vi "RT_I2C Configure.vi"(7 "Address Type (7-bit)":enum16{"7-bit", "10-bit"}(ring), 8 "error in":errorcluster, 9 "Clock Rate":u32, 10 "IICSlaveAddress":u16, 11 "FPGA VI Reference In":T1) -> (0 "error out":errorcluster, 3 "FPGA VI Reference Out":T1)   [LabVIEW 2018]
uses:
  Data Def/RT_FPGA VI Reference.ctl
  <vilib>/Utility/error.llb/Error Cluster From Error Code.vi
  <vilib>/rvi/errors/niLvFpgaAdjustHostInterfaceError.vi
  <vilib>/rvi/interface/nirviReadWriteControl/nirviReadWriteControl.xnode
  NiFpgaLv.dll
  <vilib>/rvi/interface/Simulation/niFpgaSimulationCallBeginRW.vi
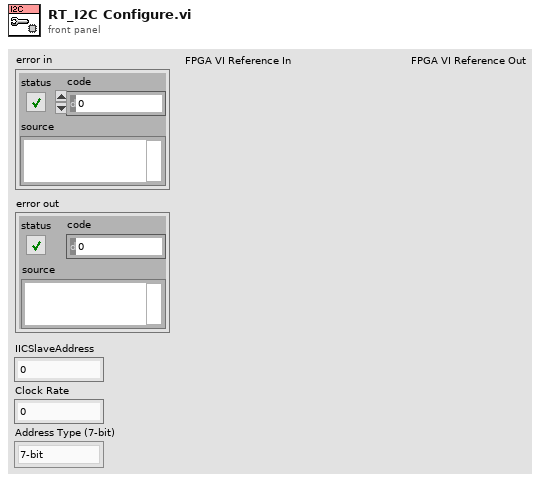
[diagram p1: front panel]
types:
  T1 = typedef "RT_FPGA VI Reference.ctl" = refnum<k20>
  T2 = cluster{"Address":u16, "Address Type (7-bit)":enum16{"7-bit", "10-bit"}, "I2C Parameters":cluster{"Clock Divider":u32}}
  T3 = enum16{"Idle", "Set Idle", "Config", "Read", "Write", "Arm", "Auto Run", "Auto Config", "Auto Write", "Auto Arm", "Auto Read", "Auto Check"}
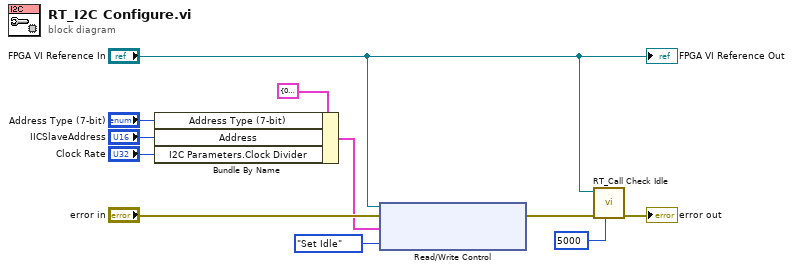
[diagram p0: block diagram]
diagram:
  n1 = Bundle By Name(cluster=T2 {"Address"=0, "Address Type (7-bit)"=enum."7-bit", "I2C Parameters"={"Clock Divider"=0}} ("I2C Protocol Configure"), "Address Type (7-bit)"="Address Type (7-bit)", "Address"="IICSlaveAddress", "I2C Parameters.Clock Divider"="Clock Rate") -> (w1:T2)
  n2 = xnode "Read/Write Control"("FPGA VI Reference In"="FPGA VI Reference In", "error in"="error in", "I2C Protocol Configure"=w1, "I2C Loop State"=T3."Set Idle") -> ("error out"=w7:errorcluster)  [unwired: 1 out]
  n3 = call "RT_Call Check Idle.vi"("Timeout?"=5000, "error in"=w7, "FPGA VI Reference In"="FPGA VI Reference In") -> ("error out"=→"error out":errorcluster)  [unwired: 7 in, 1 out]
  "FPGA VI Reference Out" <- "FPGA VI Reference In"
